vi "dbcToCan.vi"() -> ()   [LabVIEW 2023]
panel:
  out "data":string
  out "subarray":string[](array[string])
  out "serchID":i32[](array[numeric])
  out "Array 4":i32[](array[numeric])
  in  "Array 2":string[][](array[string])
  in  "Array":T1(array[cluster])
  out "vcu1Element":string
  out "id":string
  in  "canArrayDataOut":string[](array[string])
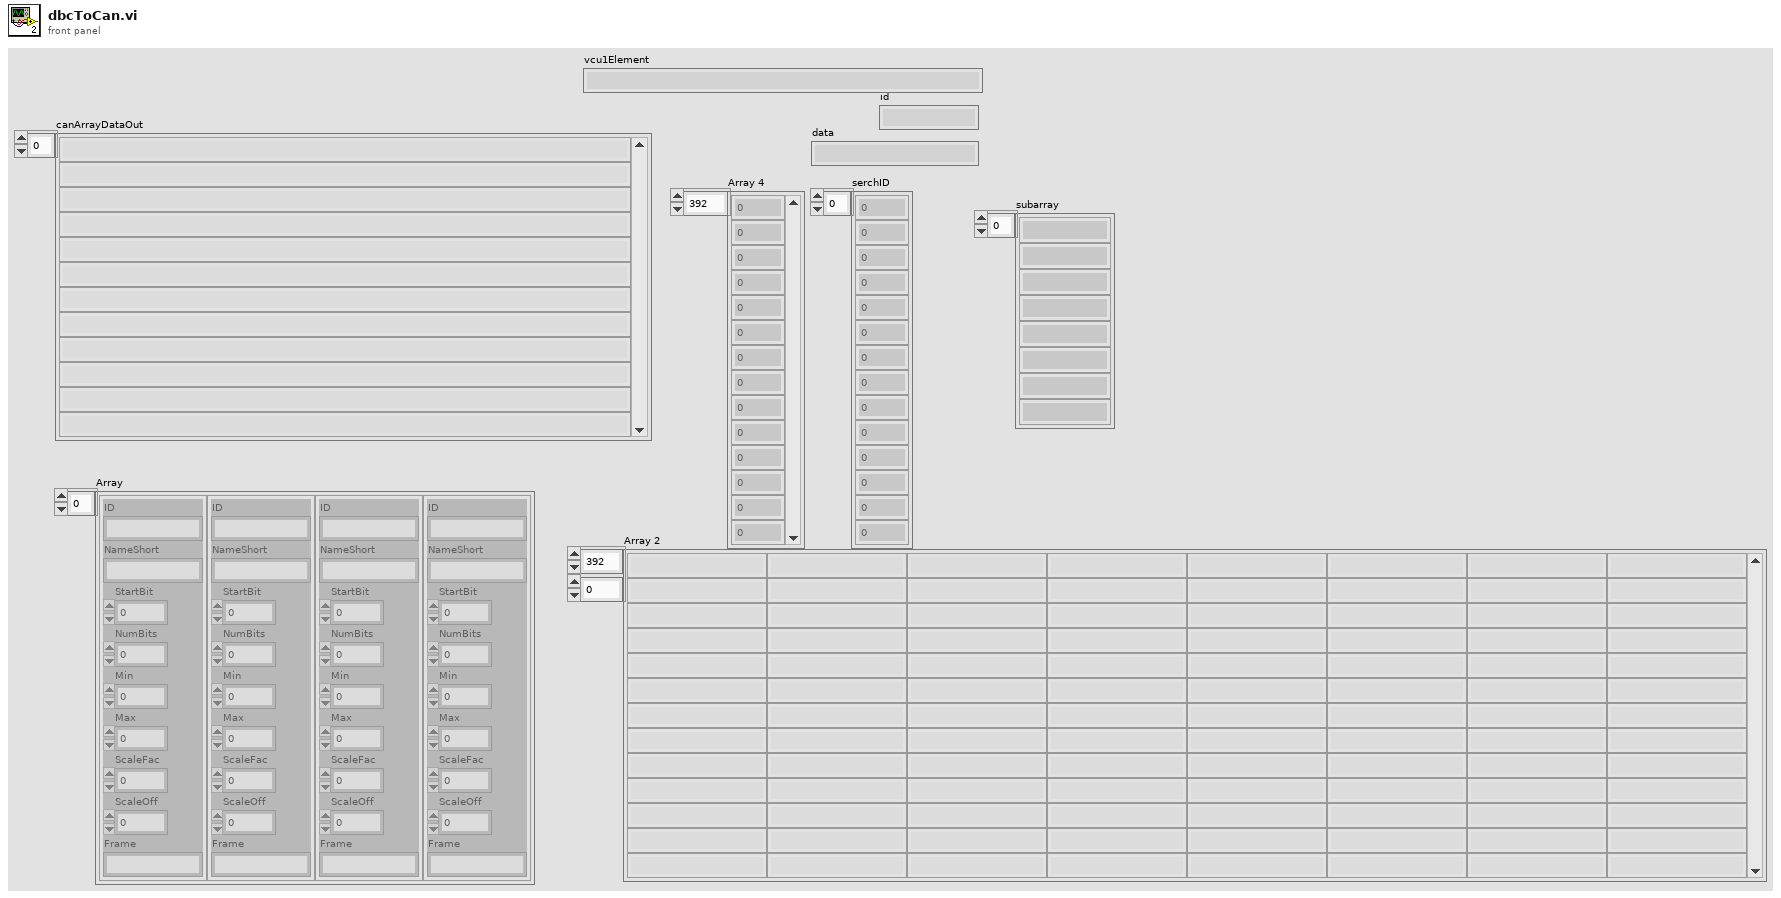
[diagram p1: front panel]
types:
  T1 = cluster{"ID":string, "NameShort":string, "StartBit":u32, "NumBits":u32, "Min":dbl, "Max":dbl, "ScaleFac":dbl, "ScaleOff":dbl, "Frame":string}[]
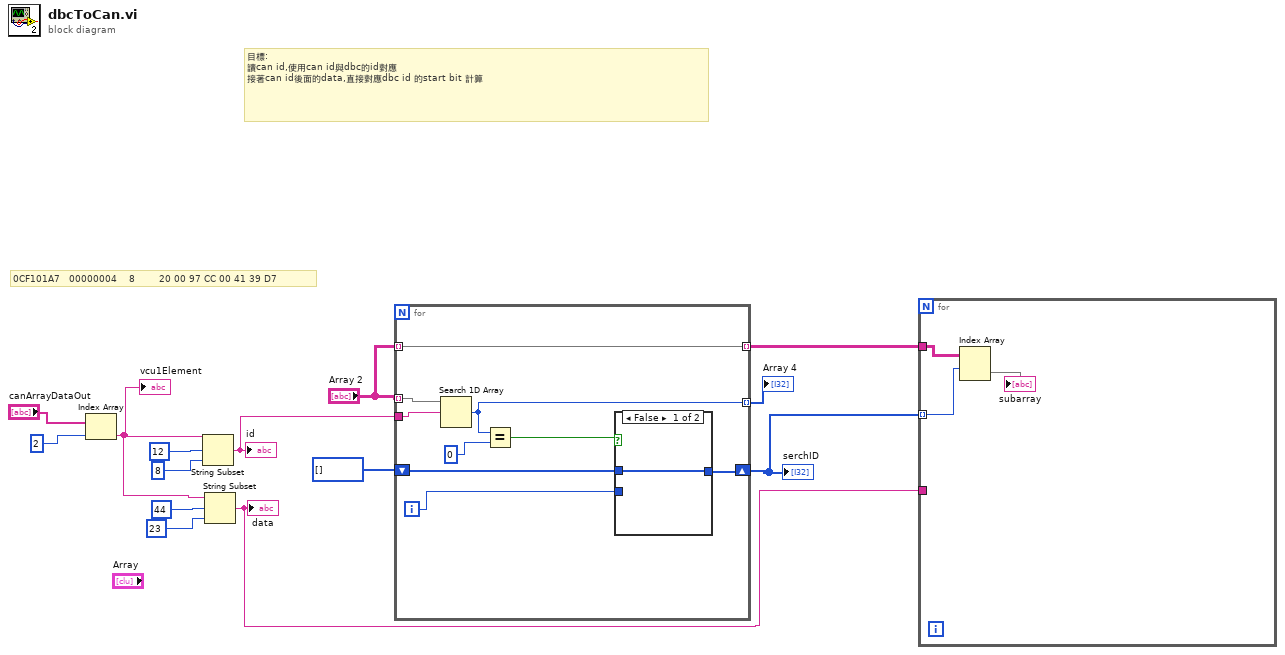
[diagram p0: block diagram]
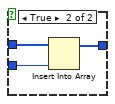
[diagram p2: hidden frame]
diagram:
  # "目標:\n讀can id,使用can id與dbc的id對應\n接著can id後面的data,直接對應dbc id 的start bit 計算"
  # "0CF101A7   00000004    8        20\t00\t97\tCC\t00\t41\t39\tD7"
  n1 = Index Array(array="canArrayDataOut", index=2) -> (element=w2:string)
  "vcu1Element" <- w2
  n2 = String Subset(string=w2, offset (0)=12 ("length (rest)"), length (rest)=8 ("length (rest)")) -> (substring=w10:string)
  "id" <- w10
  n3 = String Subset(string=w2, offset (0)=44 ("length (rest)"), length (rest)=23 ("length (rest)")) -> (substring=w1:string)
  "data" <- w1
  n4 = for {
    tunnel: "Array 2" -> [w23] mode=indexing
    tunnel: w10 -> [w22]
    tunnel: [w21] -> w9 mode=indexing
    shift-right: [w18] -> w5
    shift-left: i32[] [] -> [w16]
    tunnel: [w15] -> w6 mode=indexing
    tunnel: "Array 2" -> [w15] mode=indexing
    i -> [w17]
    n5 = Search 1D Array(1D array=w23, element=w22) -> (index of element=w21:i32)  [unwired: 1 in]
    n6 = Equal?(x=w21, y=0) -> (x = y?=w19:bool)
    n7 = case shown="False" w19 {
      tunnel: [w24 w27] -> w18
      tunnel: w17 -> [_ w26]
      tunnel: w16 -> [w24 w25]
      frame False {
      }
      frame True {
        n8 = Insert Into Array(array=w25, new element=w26) -> (w27:i32[])  [unwired: 1 in]
      }
    }
  }
  "Array 4" <- w9
  "serchID" <- w5
  n9 = for {
    tunnel: w6 -> [w30]
    tunnel: w5 -> [w29] mode=indexing
    tunnel: w1 -> [_]
    n10 = Index Array(array=w30, index (row)=w29) -> (element=→"subarray":string[])  [unwired: 1 in]
  }
